vi "ChangeColor.vi"(8 "error in (no error)":errorcluster caption="错误输入（无错误）", 9 "颜色[4]":cluster{u32, u32}[](array[cluster]), 11 "RandomMoveBool 输入":refnum<class "RandomMoveBool.lvclass">) -> (0 "error out":errorcluster caption="错误输出", 3 "RandomMoveBool 输出":refnum<class "RandomMoveBool.lvclass">)   [LabVIEW 2018, in "RandomMoveBool.lvclass"]
uses:
  RandomMoveBool.lvclass
  RandomMoveBool.lvclass/RandomMoveBool.ctl
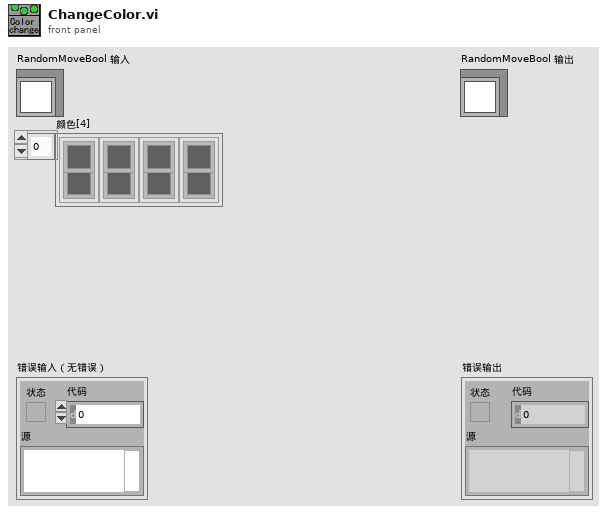
[diagram p1: front panel]
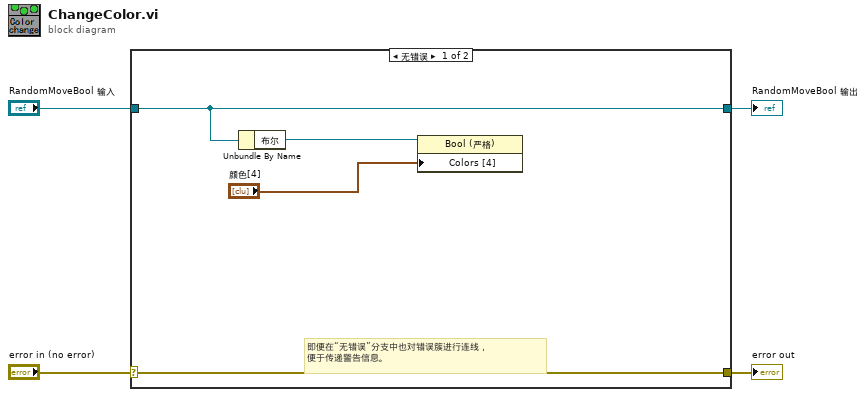
[diagram p0: block diagram]
diagram:
  n1 = case shown="无错误" "error in (no error)" {
    selector: "error in (no error)" -> [w8 w10]
    tunnel: [w8 w10] -> w3
    tunnel: [w7 w9] -> w1
    tunnel: "RandomMoveBool 输入" -> [w7 w9]
    frame No Error {
      # "即便在“无错误”分支中也对错误簇进行连线，\n便于传递警告信息。"
      n2 = Unbundle By Name(w7) -> ("布尔"=w6:refnum<vi>)
      n3 = property class="Bool (严格)"(reference=w6, "Colors [4]"="颜色[4]") -> ()  [unwired: 1 in, 2 out]
    }
    frame Error {
    }
  }
  "error out" <- w3
  "RandomMoveBool 输出" <- w1
